vi "未命名 2.vi"() -> ()   [LabVIEW 2013]
uses:
  <vilib>/gmath/NI_Gmath.lvlib
  <vilib>/Analysis/NI_AALPro.lvlib
  <vilib>/Analysis/2dsp.llb/Cross Power (DBL).vi
panel:
  in  "设备数据簇":T1={"设备型号"=enum."NAR6000", "设备配置参数"={"中心频点"=400000000, "频宽"=200000000, "RBW"=50000, "参考电平"=-50}}
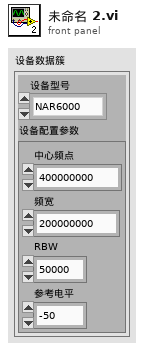
[diagram p1: front panel]
types:
  T1 = typedef "设备数据簇.ctl" = cluster{"设备型号":enum16{"NAR6000", "安捷伦"}, "设备配置参数":cluster{"中心频点":u64, "频宽":u64, "RBW":i32, "参考电平":i32}}
  T2 = cluster{"TCP地址":string, "TCP端口号":i32, "TCP网络连接引用句柄":refnum<k5>}
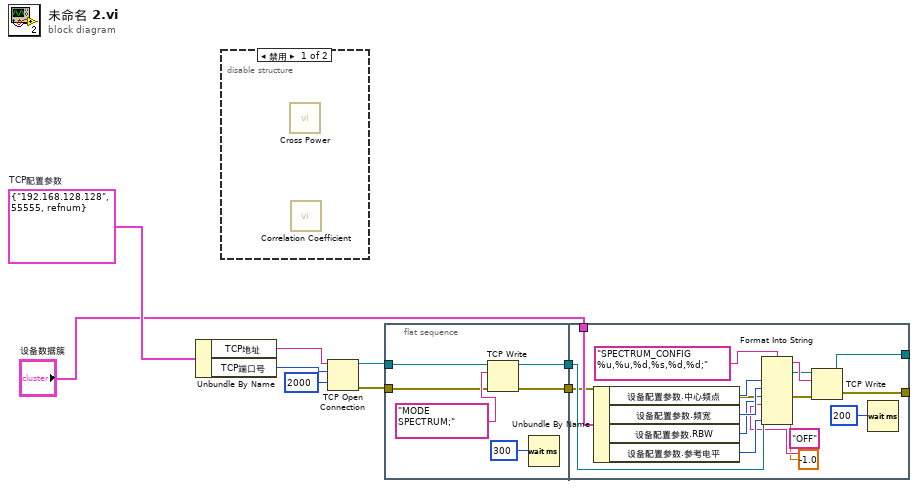
[diagram p0: block diagram]
diagram:
  w2 = T2 {"TCP地址"="192.168.128.128", "TCP端口号"=55555, "TCP网络连接引用句柄"=refnum}  # TCP配置参数
  n1 = Unbundle By Name(w2) -> ("TCP地址"=w6:string, "TCP端口号"=w5:i32)
  n2 = disable-structure shown="禁用" {
    frame Disabled {
      n3 = call-poly <vilib>:"Cross Power.vi"() -> ()  [unwired: 2 in, 2 out]
      n4 = call <vilib>:"Correlation Coefficient.vi"() -> ()  [unwired: 10 in, 2 out]
    }
    frame Enabled {
    }
  }
  n5 = TCP Open Connection ("打开TCP连接")(address=w6, remote port or service name=w5, timeout ms (60000)=2000 ("超时毫秒(60000)")) -> (connection ID=w7:refnum<k5>, error out=w4:errorcluster)  [unwired: 2 in]
  n6 = flat-sequence {
    tunnel: w7 -> [w15]
    tunnel: [w13] -> w9
    tunnel: w4 -> [w11]
    tunnel: [w10] -> w8
    tunnel: w9 -> [w26]
    tunnel: "设备数据簇" -> [w28]
    tunnel: w8 -> [w18]
    tunnel: [w17] -> _
    tunnel: [w16] -> _
    frame #0 {
      n7 = TCP Write(connection ID=w15, data in="MODE SPECTRUM;" ("指令"), error in (no error)=w11) -> (connection ID out=w13:refnum<k5>, error out=w10:errorcluster)  [unwired: 1 in, 1 out]
      n8 = Wait (ms)(milliseconds to wait=300) -> ()  [unwired: 1 out]
    }
    frame #1 {
      n9 = Unbundle By Name(w28) -> ("设备配置参数.中心频点"=w25:u64, "设备配置参数.频宽"=w24:u64, "设备配置参数.RBW"=w23:i32, "设备配置参数.参考电平"=w22:i32)
      n10 = Format Into String(format string="SPECTRUM_CONFIG %u,%u,%d,%s,%d,%d;" ("指令"), w25, w24, w23, "OFF" ("输入 4"), -1.0 ("输入 5"), w22) -> (resulting string=w27:string)  [unwired: 2 in, 1 out]
      n11 = TCP Write(connection ID=w26, data in=w27, error in (no error)=w18) -> (connection ID out=w16:refnum<k5>, error out=w17:errorcluster)  [unwired: 1 in, 1 out]
      n12 = Wait (ms)(milliseconds to wait=200) -> ()  [unwired: 1 out]
    }
  }
